vi "Pass.vi"(8 "error in (no error)":errorcluster, 11 "Constraint in":refnum<class "Constraint.lvclass">) -> (0 "error out":errorcluster, 3 "Constraint out":refnum<class "Constraint.lvclass">)   [LabVIEW 2017, in "Constraint.lvlib" / "Constraint.lvclass"]
doc: "Reports a successful test."
uses:
  Constraint.lvclass
  Framework/LVUnit Test Framework/LVUnit Test Framework.lvclass
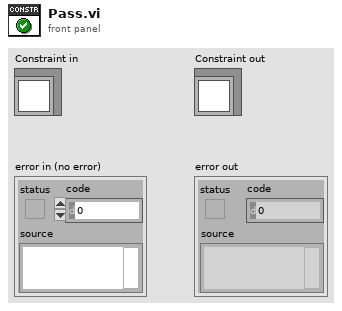
[diagram p1: front panel]
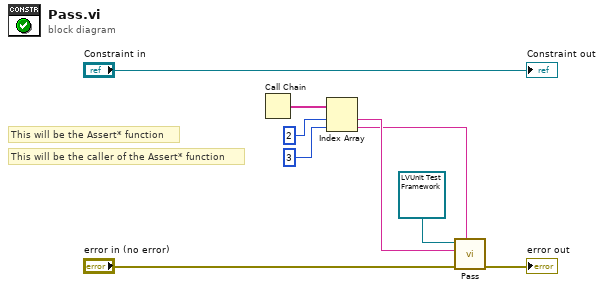
[diagram p0: block diagram]
diagram:
  # "This will be the Assert* function"
  # "This will be the caller of the Assert* function"
  n1 = Call Chain() -> (call chain=w5:string[])
  n2 = Index Array(array=w5, index #1=2 ("index"), index #2=3 ("index")) -> (element #1=w2:string, element #2=w1:string)
  n3 = call-dynamic "Pass.vi"("Caller"=w1, "error in (no error)"="error in (no error)", "Assertion"=w2, "Test Framework in"=refnum<class "LVUnit Test Framework.lvclass"> refnum ("Framework.lvlib:LVUnit Test Framework.lvclass")) -> ("error out"=→"error out":errorcluster)  [unwired: 6 in, 1 out]
  "Constraint out" <- "Constraint in"
